vi "seven-segment-display-2.vi"() -> ()   [LabVIEW 2014]
uses:
  <vilib>/Utility/miscctls.llb/LVMinMaxIncTypeDef.ctl
panel:
  out "seven segment":T1
  in  "stop":bool
  in  "Input":i32 min=0 max=9
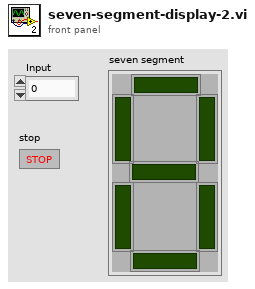
[diagram p1: front panel]
types:
  T1 = cluster{"a":bool, "b":bool, "c":bool, "d":bool, "e":bool, "f":bool, "g":bool}
  T2 = typedef "LVMinMaxIncTypeDef.ctl" = cluster{"Minimum":dbl, "Maximum":dbl, "Increment":dbl}
  T3 = cluster{"Boolean array[0]":bool, "Boolean array[1]":bool, "Boolean array[2]":bool, "Boolean array[3]":bool, "Boolean array[4]":bool, "Boolean array[5]":bool, "Boolean array[6]":bool}
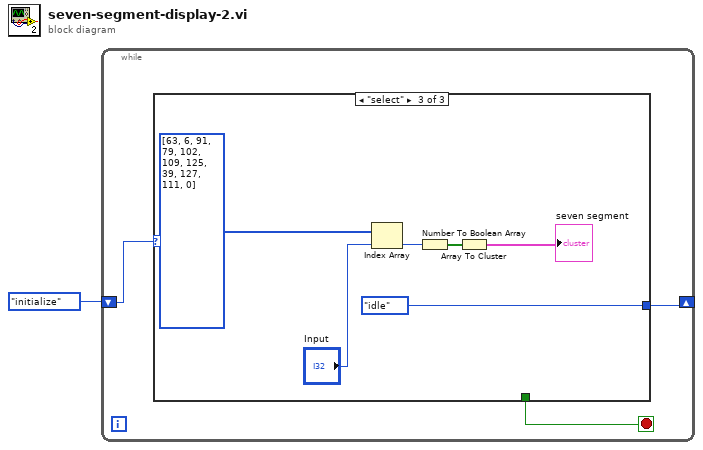
[diagram p0: block diagram]
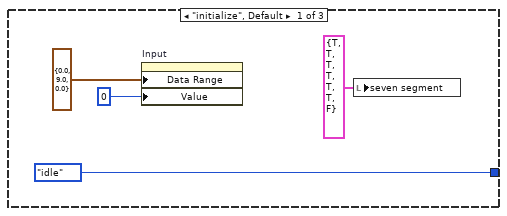
[diagram p2: hidden frame]
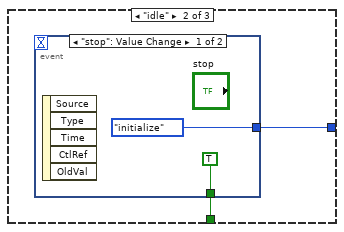
[diagram p3: hidden frame]
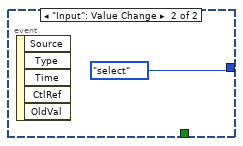
[diagram p4: hidden frame]
diagram:
  n1 = while {
    shift-right: [w3] -> _
    shift-left: enum16{"initialize", "idle", "select"}."initialize" -> [w4]
    stop <- w2 stop-if-true
    n2 = case shown="\"select\"" w4 {
      tunnel: [enum16{"initialize", "idle", "select"}."idle" w10 enum16{"initialize", "idle", "select"}."idle"] -> w3
      tunnel: [_ w9 _] -> w2
      frame "initialize", Default {
        n3 = property on="Input" class="DigNum (strict)"("Data Range"=T2 {"Minimum"=0.0, "Maximum"=9.0, "Increment"=0.0} ("Data Entry Limits"), "Value"=0) -> ()  [unwired: 2 in, 2 out]
        n4 = local write "seven segment"(T1 {"a"=TRUE, "b"=TRUE, "c"=TRUE, "d"=TRUE, "e"=TRUE, "f"=TRUE, "g"=FALSE} ("seven segment")) -> ()
      }
      frame "idle" {
        n5 = event shown="[0] \"stop\": Value Change" {
          selector: _ -> [_ _]
          dyn-events: _ -> [_ _]
          timeout: _ -> [_ _]
          tunnel: [enum16{"initialize", "idle", "select"}."initialize" enum16{"initialize", "idle", "select"}."select"] -> w10
          tunnel: [TRUE _] -> w9
          event "stop": Value Change {
            n6 = event-data() -> ()  [unwired: 1 in, 5 out]
          }
          event "Input": Value Change {
            n7 = event-data() -> ()  [unwired: 1 in, 5 out]
          }
        }
      }
      frame "select" {
        n8 = Index Array(array=i32[] [63, 6, 91, 79, 102, 109, 125, 39, 127, 111, 0], index="Input") -> (element=w16:i32)
        n9 = Number To Boolean Array(number=w16) -> (Boolean array=w15:bool[])
        n10 = Array To Cluster(array=w15) -> (cluster=→"seven segment":T3)
      }
    }
  }
